vi "cuda_dll_test main.vi"() -> ()   [LabVIEW 2017]
uses:
  <vilib>/vision/NI_Vision_Development_Module.lvlib
panel:
  out "rdp profile":sgl[][](graph)
  in  "stop":bool
  out "rdp_mean":sgl[][](graph)
  out "rdp_mean out":sgl[][](array[numeric])
  out "yc out":sgl[](array[numeric])
  out "xc out":sgl[](array[numeric])
  out "rdp_profile out":sgl[][](array[numeric])
  in  "sampling rate":i32=5
  out "y_qi_out":sgl[][](array[numeric])
  out "x_qi_out":sgl[][](array[numeric])
  out "rdp_profile":sgl[][][](array[numeric])
  out "Image":T1(plugin-control)
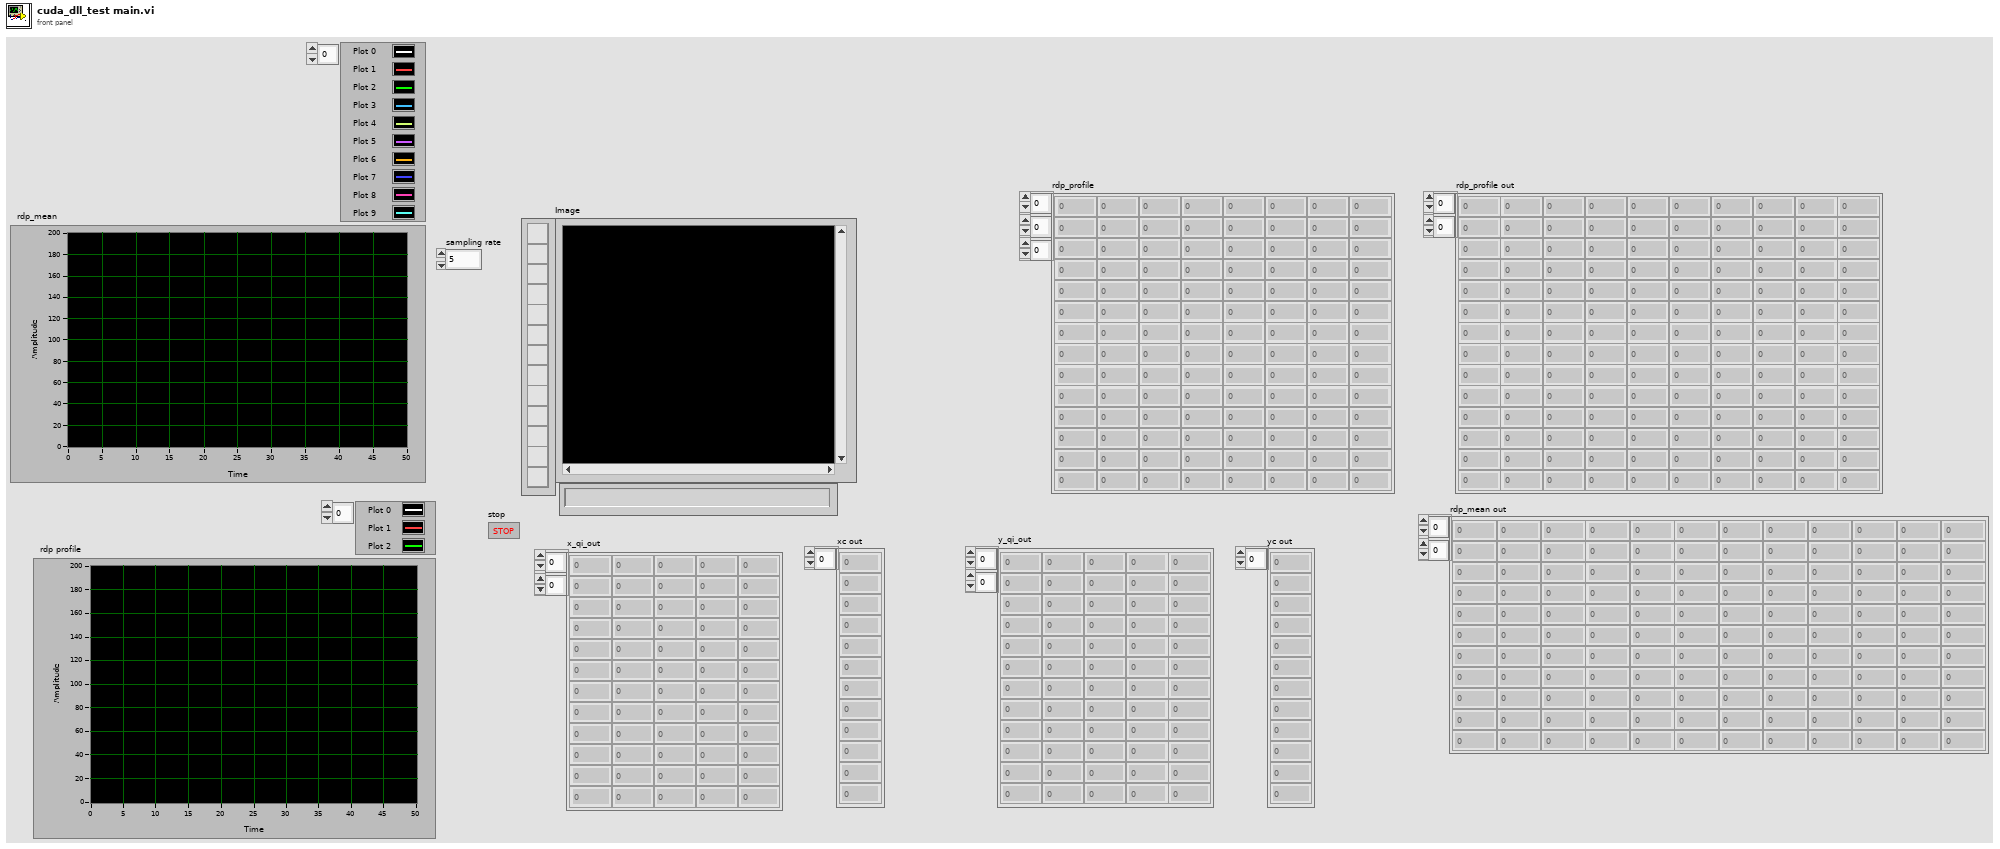
[diagram p1: front panel]
types:
  T1 = typedef "IMAQ Image.ctl" = refnum<image>
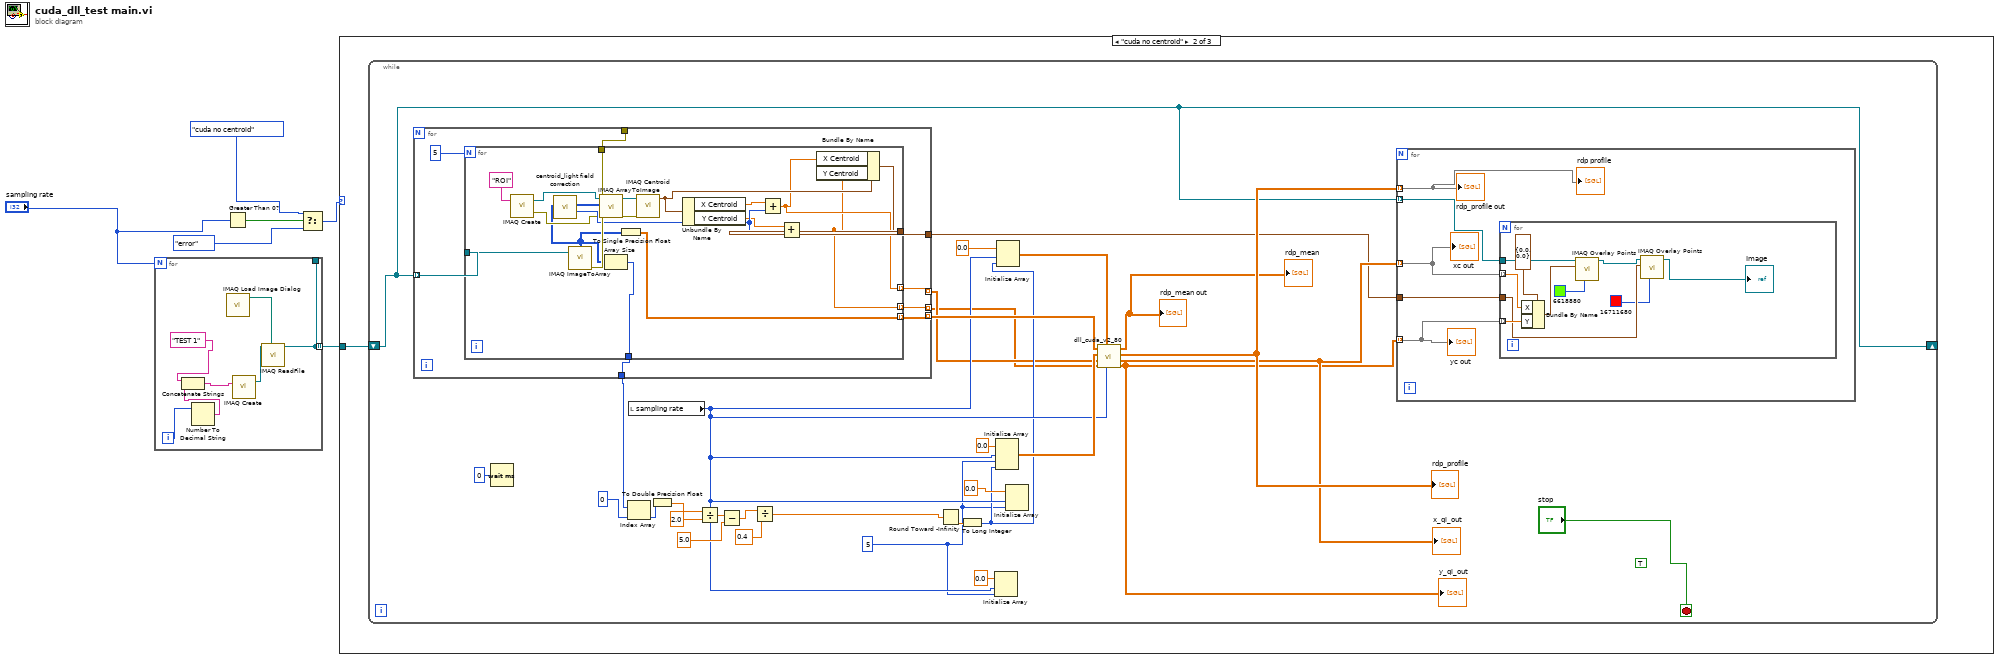
[diagram p0: block diagram]
diagram:
  n1 = for {
    N: "sampling rate" -> [_]
    tunnel: [w12] -> _
    tunnel: [w12] -> w6 mode=indexing
    i -> [w9]
    n2 = Number To Decimal String(number=w9) -> (decimal integer string=w8:string)  [unwired: 1 in]
    n3 = Concatenate Strings("TEST 1" ("Image Name"), w8) -> (w7:string)
    n4 = call "IMAQ Load Image Dialog"() -> ("Path"=w11:path)  [unwired: 9 in, 2 out]
    n5 = call "IMAQ Create"("Image Name"=w7) -> ("New Image"=w13:T1)  [unwired: 4 in, 1 out]
    n6 = call "IMAQ ReadFile"("File Path"=w11, "Image"=w13) -> ("Image Out"=w12:T1)  [unwired: 5 in, 4 out]
  }
  n7 = Greater Than 0?(x="sampling rate") -> (x > 0?=w4:bool)
  n8 = Select(t=enum16{"cuda", "cuda no centroid", "error"}."cuda no centroid", s=w4, f=enum16{"cuda", "cuda no centroid", "error"}."error") -> (s? t:f=w1:enum16{"cuda", "cuda no centroid", "error"})
  n9 = case shown="\"cuda no centroid\"" w1 {
    tunnel: w6 -> [_ w14 _]
    frame "cuda", Default {
    }
    frame "cuda no centroid" {
      n10 = while {
        shift-right: [w16] -> _
        shift-left: w14 -> [w16]
        stop <- "stop" stop-if-true
        (unwired) TRUE
        w24 = 5 ("n_frame")
        n11 = for {
          tunnel: w16 -> [w64] mode=indexing
          tunnel: [w67] -> w33
          tunnel: [w66] -> w31 mode=indexing
          tunnel: [w65] -> _
          tunnel: [w63] -> w21
          tunnel: [w62] -> w20 mode=indexing
          tunnel: [w61] -> w19 mode=indexing
          n12 = for {
            N: 5 -> [_]
            tunnel: w64 -> [w86]
            tunnel: [w85] -> w67
            tunnel: [w84] -> w66 mode=indexing
            tunnel: [w83] -> w65
            tunnel: [w72] -> w63
            tunnel: [w70] -> w62 mode=indexing
            tunnel: [w69] -> w61 mode=indexing
            n13 = call "IMAQ Create"("Image Name"="ROI") -> ("New Image"=w77:T1, "error out"=w78:errorcluster)  [unwired: 4 in]
            n14 = call "IMAQ ImageToArray"("Image"=w86) -> ("error out"=w83:errorcluster, "Image Pixels (U8)"=w71:u8[][])  [unwired: 3 in, 3 out]
            n15 = call "centroid_light field correction.vi"("ROI array (no trans)"=w71) -> ("xybase core"=w81:i32, "ROI array out"=w74:u8[][])  [unwired: 9 in]
            n16 = call "IMAQ ArrayToImage"("error in (no error)"=w78, "Image Pixels (U8)"=w74, "Image"=w77) -> ("error out"=w76:errorcluster, "Image Out"=w75:T1)  [unwired: 7 in]
            n17 = Array Size(array=w71) -> (size(s)=w85:i32[])
            n18 = To Single Precision Float(number=w71) -> (single precision float=w84:sgl[][])
            n19 = call "IMAQ Centroid"("error in (no error)"=w76, "Image"=w75) -> ("Centroid"=w82:cluster{"X Centroid":sgl, "Y Centroid":sgl})  [unwired: 2 in, 1 out]
            n20 = Unbundle By Name(w82) -> ("X Centroid"=w79:sgl, "Y Centroid"=w80:sgl)
            n21 = Add(x=w79, y=w81) -> (x+y=w70:sgl)
            n22 = Add(x=w80, y=w81) -> (x+y=w69:sgl)
            n23 = Bundle By Name(cluster=w82, "X Centroid"=w70, "Y Centroid"=w69) -> (w72:cluster{"X Centroid":sgl, "Y Centroid":sgl})
          }
        }
        n24 = Wait (ms)(milliseconds to wait=u32 0) -> ()  [unwired: 1 out]
        n25 = Index Array(array=w33, index=0) -> (element=w22:i32)
        n26 = local read "sampling rate"() -> (w26:i32)
        n27 = To Double Precision Float(number=w22) -> (double precision float=w45:dbl)
        n28 = Divide(x=w45, y=2.0) -> (x/y=w44:dbl)
        n29 = Subtract(x=w44, y=5.0) -> (x-y=w43:dbl)
        n30 = Divide(x=w43, y=0.4) -> (x/y=w42:dbl)
        n31 = Round Toward -Infinity(1:w42) -> (0:w41:dbl)
        n32 = To Long Integer(number=w41) -> (32bit integer=w25:i32)
        n33 = Initialize Array(sgl 0.0 ("element"), w26, w24) -> ()  [unwired: 1 out]
        n34 = Initialize Array(sgl 0.0 ("element"), w26, w24, w25) -> (w36:sgl[][][])
        n35 = Initialize Array(sgl 0.0 ("element"), w26, w25) -> (w18:sgl[][])
        n36 = Initialize Array(sgl 0.0 ("element"), w26, w24) -> ()  [unwired: 1 out]
        n37 = call "dll_cuda_v2_80.vi"("n_stream"=w26, "rdp_mean"=w18, "yc"=w19, "xc"=w20, "rdp_profile"=w36, "img_mat 4d"=w31) -> ("yc out"=w27:sgl[][], "xc out"=w28:sgl[][], "rdp_profile out"=w29:sgl[][][], "rdp_mean out"=→"rdp_mean out" →"rdp_mean":sgl[][])  [unwired: 2 in]
        "rdp_profile" <- w29
        "y_qi_out" <- w27
        "x_qi_out" <- w28
        n38 = for {
          tunnel: w29 -> [w47] mode=indexing
          tunnel: w28 -> [w50] mode=indexing
          tunnel: w27 -> [w49] mode=indexing
          tunnel: w21 -> [w48]
          tunnel: w16 -> [w46] mode=indexing
          n39 = for {
            tunnel: w46 -> [w59]
            tunnel: w50 -> [w57] mode=indexing
            tunnel: w49 -> [w56] mode=indexing
            tunnel: w48 -> [w53]
            n40 = Bundle By Name(cluster=cluster{"X":sgl, "Y":sgl} {"X"=0.0, "Y"=0.0} ("Point"), "X"=w57, "Y"=w56) -> (w55:cluster{"X":sgl, "Y":sgl})
            n41 = call "IMAQ Overlay Points"("Color"=u32 6618880, "Point"=w55, "Image"=w59) -> ("Image Out"=w54:T1)  [unwired: 7 in, 1 out]
            n42 = call "IMAQ Overlay Points"("Color"=u32 16711680, "Point"=w53, "Image"=w54) -> ("Image Out"=→"Image":T1)  [unwired: 7 in, 1 out]
          }
          "rdp_profile out" <- w47
          "xc out" <- w50
          "yc out" <- w49
          "rdp profile" <- w47
        }
      }
    }
    frame "error" {
    }
  }
